vi "Configure FFT Measurement Trigger Offset.vi"(5 "Fixed Offset (0.1e-3)":dbl=0.0001 format="%^.3e", 6 "Variable Offset Stop (1E-3)":dbl=0.001 format="%^.3e", 7 "Variable Offset Start (0.0)":dbl format="%^.3e", 8 "error in (no error)":errorcluster, 9 "Offset Mode (Fixed)":i32(ring) items=["Fixed", "Variable"], 10 "Instance (1)":i32=1, 11 "VISA resource name":refnum<visa-resource-name>) -> (0 "error out":errorcluster, 3 "VISA resource name out":refnum<visa-resource-name>)   [LabVIEW 2020, in "Rohde&Schwarz CMXP GPRF.lvlib"]
doc: "Selects fixed or variable trigger offset. In the \"FFT Spectrum Analyzer\" measurement, the trigger offset defines the center of the FFT window.\n\nAttributes:\nRSCMXPGPRF_ATTR_FFT_MEASUREMENT_TRIGGER_OFFSET_MODE\nRSCMXPGPRF_ATTR_FFT_MEASUREMENT_TRIGGER_OFFSET\n\nRemote-control commands:\nTRIGger:GPRF:MEAS<i>:FFTSanalyzer:OMODe\nTRIGger:GPRF:MEAS<i>:FFTSanalyzer:OSSTop\nTRIGger:GPRF:MEAS<i>:FFTSanalyzer:OFFSet"
uses:
  <instrlib>/Rohde&Schwarz CMXP GPRF/Rohde&Schwarz CMXP GPRF.lvlib
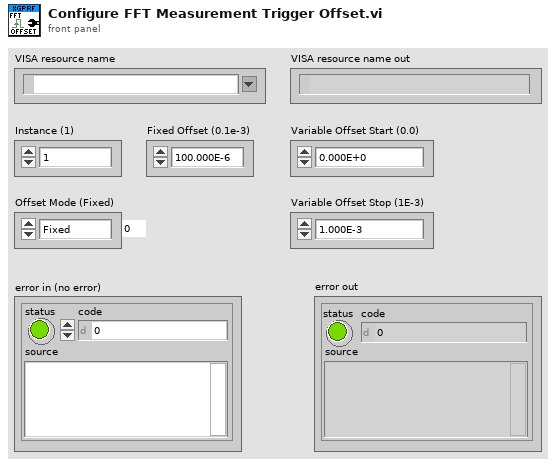
[diagram p1: front panel]
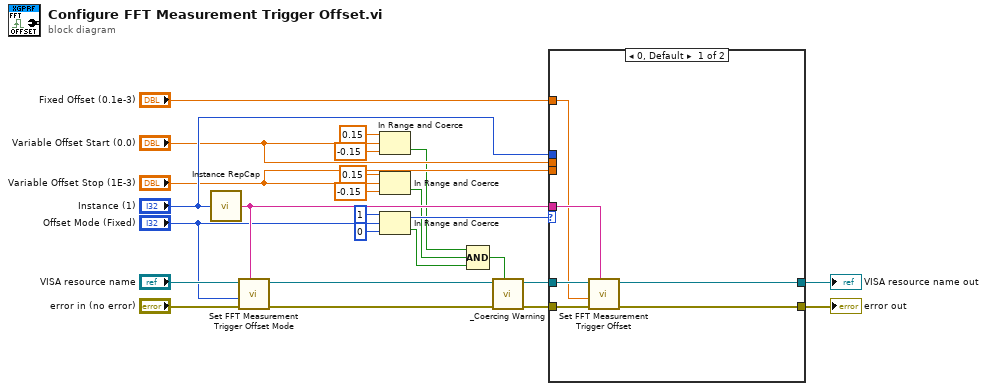
[diagram p0: block diagram]
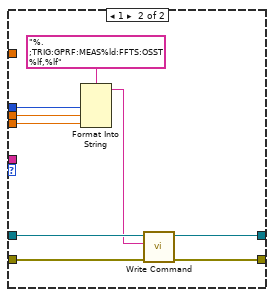
[diagram p2: hidden frame]
diagram:
  n1 = call <instrlib>:"Instance RepCap.vi"("Instance in"="Instance (1)") -> ("Instance out"=w6:string)
  n2 = call "Set FFT Measurement Trigger Offset Mode"("Repeated Capabilities"=w6, "error in (no error)"="error in (no error)", "FFT Measurement Trigger Offset Mode (0 - Fixed)"="Offset Mode (Fixed)", "instrument handle"="VISA resource name") -> ("error out"=w21:errorcluster, "instrument handle out"=w20:refnum<visa-resource-name>)  [unwired: 6 in]
  n3 = In Range and Coerce(upper limit=0.15, x="Variable Offset Start (0.0)", lower limit=-0.15) -> (In Range?=w1:bool)  [unwired: 1 out]
  n4 = In Range and Coerce(upper limit=0.15, x="Variable Offset Stop (1E-3)", lower limit=-0.15) -> (In Range?=w2:bool)  [unwired: 1 out]
  n5 = In Range and Coerce(upper limit=1, x="Offset Mode (Fixed)", lower limit=0) -> (coerced(x)=w5:i32, In Range?=w3:bool)
  n6 = Compound Arithmetic op=AND(w1, w2, w3) -> (w13:bool)
  n7 = call <instrlib>:"_Coercing Warning.vi"("In Range?"=w13, "error in (no error)"=w21, "VISA resource name"=w20) -> ("error out"=w22:errorcluster, "VISA resource name out"=w23:refnum<visa-resource-name>)  [unwired: 7 in]
  n8 = case shown="0, Default" w5 {
    tunnel: w23 -> [w28 w39]
    tunnel: w22 -> [w31 w38]
    tunnel: "Instance (1)" -> [_ w37]
    tunnel: "Variable Offset Start (0.0)" -> [_ w36]
    tunnel: "Variable Offset Stop (1E-3)" -> [_ w35]
    tunnel: [w30 w34] -> w9
    tunnel: [w29 w33] -> w8
    tunnel: "Fixed Offset (0.1e-3)" -> [w26 _]
    tunnel: w6 -> [w27 _]
    frame 0, Default {
      n9 = call "Set FFT Measurement Trigger Offset"("Repeated Capabilities"=w27, "error in (no error)"=w31, "FFT Measurement Trigger Offset (0.0)"=w26, "instrument handle"=w28) -> ("error out"=w30:errorcluster, "instrument handle out"=w29:refnum<visa-resource-name>)  [unwired: 6 in]
    }
    frame 1 {
      n10 = Format Into String(format string="%.;TRIG:GPRF:MEAS%ld:FFTS:OSST %lf,%lf", w37, w36, w35) -> (resulting string=w32:string)  [unwired: 2 in, 1 out]
      n11 = call <instrlib>:"Write Command.vi"("error in (no error)"=w38, "Command"=w32, "VISA resource name"=w39) -> ("error out"=w34:errorcluster, "VISA resource name out"=w33:refnum<visa-resource-name>)  [unwired: 7 in]
    }
  }
  "error out" <- w9
  "VISA resource name out" <- w8
